vi "Grab and Attributes Setup.vi"() -> ()   [LabVIEW 2011]
doc: "The Grab and Attributes Setup example VI allows the user to view the current attributes and settings, update attribute settings, acquire images continuously, and display the images in an image control."
uses:
  <vilib>/vision/driver/NI_Vision_Acquisition_Software.lvlib
  <vilib>/vision/driver/IMAQdx.llb/IMAQdx Acquisition Mode.ctl
  <vilib>/vision/driver/IMAQdx.llb/IMAQdx Buffer Number Mode.ctl
panel:
  in  "Tab Control":T1(tab)
  in  "U32 Value Control":u32(slide) scale=0.0..4047.0
  in  "DBL Value Control":dbl(slide) min=1e-06 max=1000.0 step=1.0 scale=1e-06..1000.0
  in  "String Value Control":string
  in  "Enum Value Control":u32(ring) items=["Red", "Green", "Blue"]
  in  "Boolean Value Control":bool
  in  "Command Value Control":bool
  in  "Grab":bool
  out "Tooltip":string
  out "Units":string
  in  "Attribute Tree":string(tree)
  out "Frame Rate":dbl(knob) scale=0.0..100.0
  out "Image":T2(plugin-control)
  out "Buffer Number":u32
  in  "Camera Name":refnum<k21> caption="IMAQdx Session"
  in  "Stop":bool
  # "Overview: Demonstrates how to view the current attributes and settings, update attribute settings, acquire images continuously, and display the images in an image control.\nRequirements: Vision Acquisition Software\nInstructions: \n1. Select the Camera Name\n2. Run the VI"
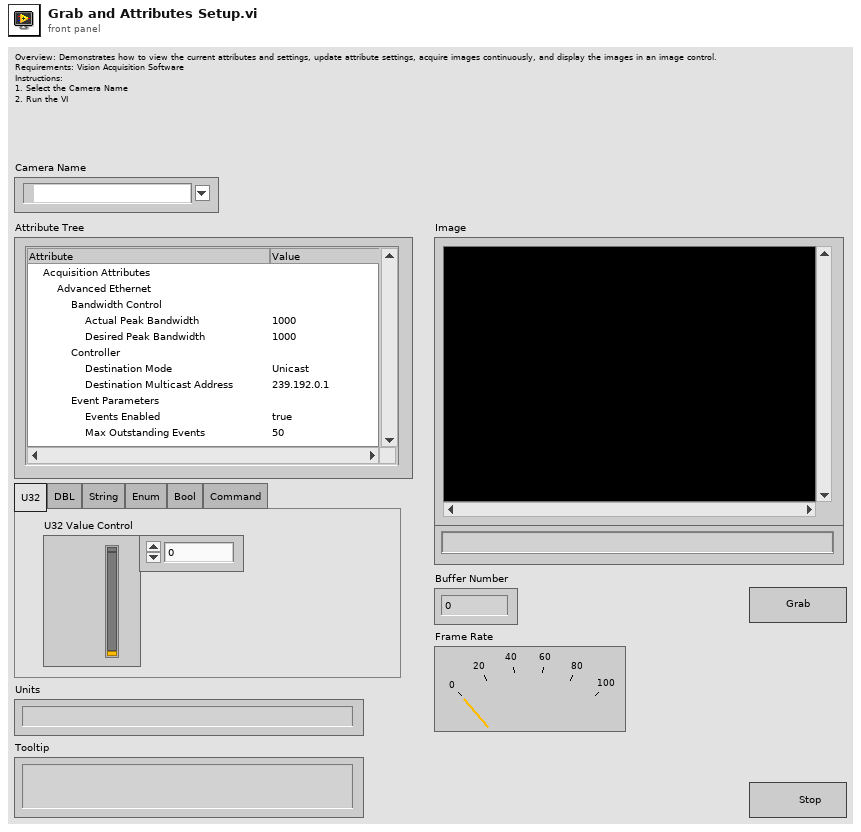
[diagram p1: front panel]
types:
  T1 = enum32{"U32", "DBL", "String", "Enum", "Bool", "Command"}
  T2 = typedef "IMAQ Image.ctl" = refnum<image>
  T3 = typedef "NI_Vision_Acquisition_Software.lvlib/IMAQdx Acquisition Mode.ctl" = enum32{"One Shot", "Continuous"}
  T4 = typedef "IMAQdx.ctl" = refnum<k21>
  T5 = cluster{"Tab Control":refnum<vi>, "U32 Value Control":refnum<vi>, "DBL Value Control":refnum<vi>, "String Value Control":refnum<vi>, "Enum Value Control":refnum<vi>, "Boolean Value Control":refnum<vi>, "Command Value Control":refnum<vi>}
  T6 = typedef "NI_Vision_Acquisition_Software.lvlib/IMAQdx Buffer Number Mode.ctl" = enum32{"Next", "Last", "Buffer Number", "Every", "Last New"}
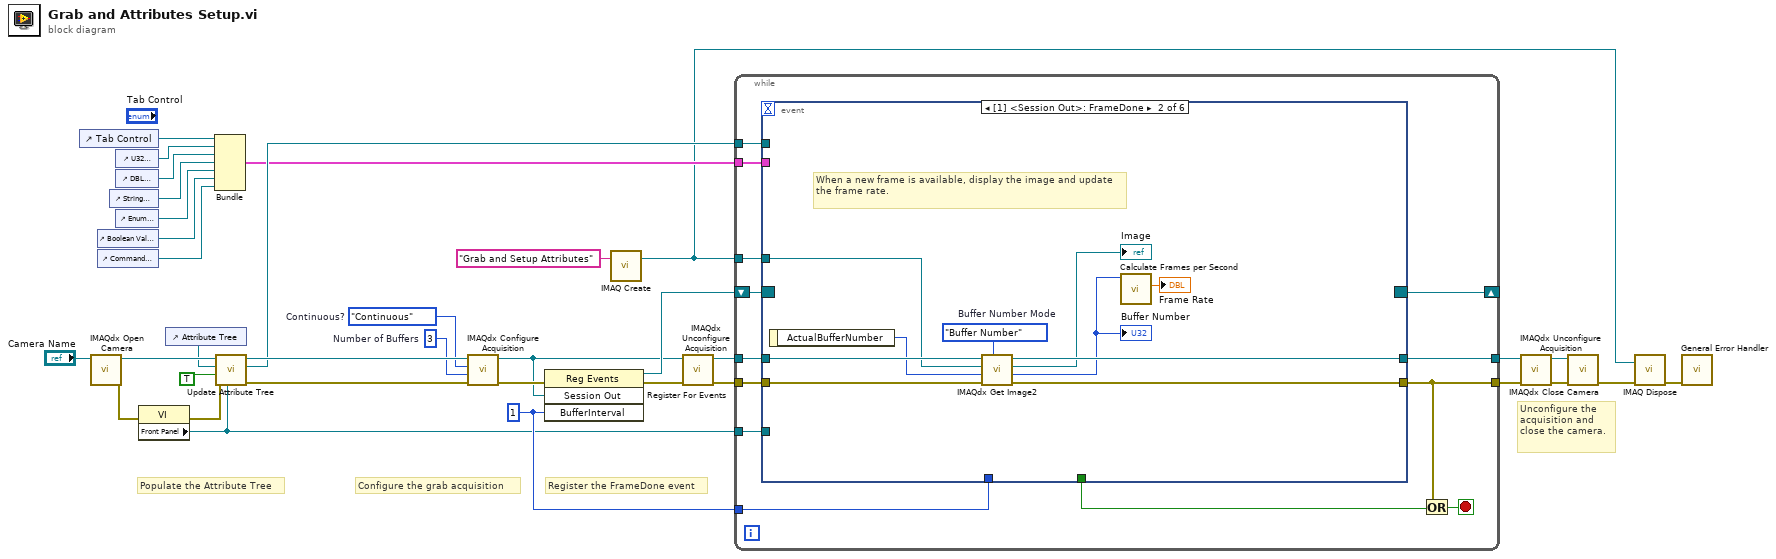
[diagram p0: block diagram]
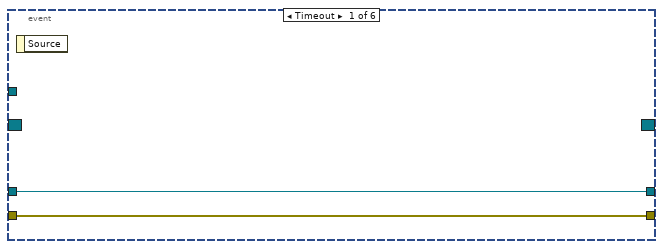
[diagram p2: hidden frame]
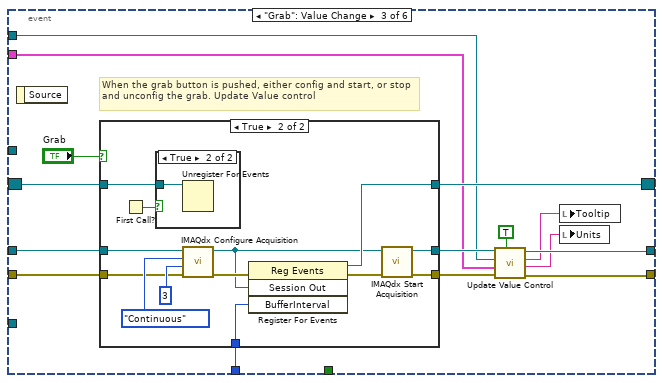
[diagram p3: hidden frame]
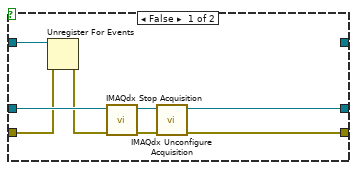
[diagram p4: hidden frame]
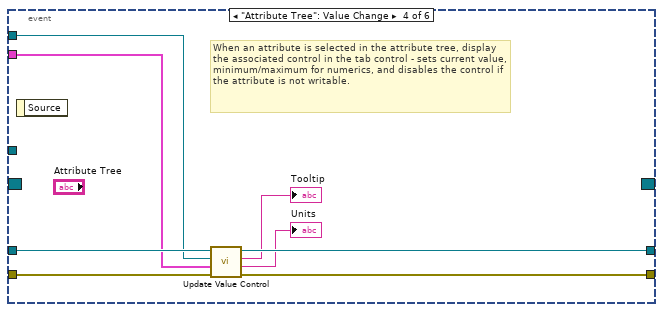
[diagram p6: hidden frame]
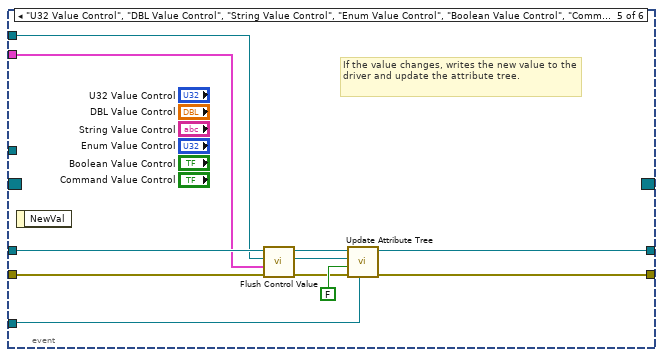
[diagram p7: hidden frame]
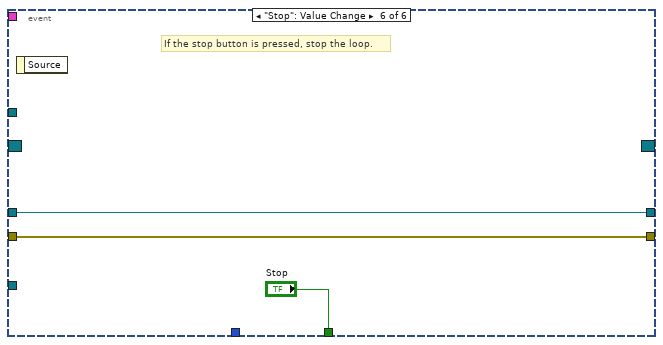
[diagram p8: hidden frame]
diagram:
  w16 = u32 1 ("BufferInterval")
  w2 = u32 3  # Number of Buffers
  w1 = IMAQdx_Acquisition_Mode."Continuous"  # Continuous?
  # "Unconfigure the acquisition and close the camera."
  # "Register the FrameDone event"
  # "Configure the grab acquisition"
  # "Populate the Attribute Tree"
  n1 = control-ref of="Tab Control"() -> (w6:refnum<vi>)
  n2 = call <vilib>:"IMAQdx Open Camera.vi"("Session In"="Camera Name") -> ("error out"=w19:errorcluster, "Session Out"=w24:T4)  [unwired: 2 in, 7 out]
  n3 = control-ref of="Boolean Value Control"() -> (w26:refnum<vi>)
  n4 = control-ref of="Command Value Control"() -> (w25:refnum<vi>)
  n5 = control-ref of="String Value Control"() -> (w30:refnum<vi>)
  n6 = control-ref of="U32 Value Control"() -> (w29:refnum<vi>)
  n7 = control-ref of="DBL Value Control"() -> (w28:refnum<vi>)
  n8 = control-ref of="Enum Value Control"() -> (w27:refnum<vi>)
  n9 = property class="VI"(error in=w19) -> (error out=w5:errorcluster, "Front Panel"=w3:refnum<vi>)  [unwired: 1 in, 1 out]
  n10 = control-ref of="Attribute Tree"() -> (w22:refnum<vi>)
  n11 = Bundle("Tab Control"=w6, "U32 Value Control"=w29, "DBL Value Control"=w28, "String Value Control"=w30, "Enum Value Control"=w27, "Boolean Value Control"=w26, "Command Value Control"=w25) -> (w11:T5)  [unwired: 1 out]
  n12 = call "Update Attribute Tree.vi"("Panel Refnum In"=w3, "error in"=w5, "Flush Tree?"=TRUE, "Tree Control In"=w22, "Camera Name In"=w24) -> ("error out"=w4:errorcluster, "Tree Control Out"=w20:refnum<vi>, "Session Out"=w23:T4)  [unwired: 4 in]
  n13 = call <vilib>:"IMAQdx Configure Acquisition.vi"("error in"=w4, "Number of Buffers"=w2, "Continuous?"=w1, "Session In"=w23) -> ("error out"=w32:errorcluster, "Session Out"=w13:T4)  [unwired: 6 out]
  n14 = register-events(error in=w32, w13, w16) -> (reference out=w31:refnum<event-registration>, error out=w15:errorcluster)  [unwired: 1 in]
  n15 = call "IMAQ Create"("Image Name"="Grab and Setup Attributes") -> ("New Image"=w8:T2)  [unwired: 3 in, 2 out]
  n16 = call <vilib>:"IMAQdx Unconfigure Acquisition.vi"("error in"=w15, "Session In"=w13) -> ("error out"=w14:errorcluster, "Session Out"=w12:T4)  [unwired: 8 out]
  n17 = while {
    tunnel: [w44] -> w18
    tunnel: w14 -> [w46]
    tunnel: w12 -> [w47]
    tunnel: [w37] -> w17
    tunnel: w8 -> [w45]
    tunnel: w20 -> [w42]
    tunnel: w3 -> [w41]
    tunnel: w16 -> [w39]
    shift-right: [w38] -> _
    shift-left: w31 -> [w43]
    tunnel: w11 -> [w36]
    stop <- w48 stop-if-true
    n18 = event shown="[1] <Session Out>: FrameDone" {
      selector: w43 -> [_ _ w71 _ _ _]
      dyn-events: [_ _ w73 _ _ _] -> w38
      timeout: _ -> [_ _ _ _ _ _]
      tunnel: w47 -> [w49 w60 w75 w105 w115 w117]
      tunnel: w46 -> [w50 w59 w70 w103 w116 w118]
      tunnel: w45 -> [_ w58 _ _ _ _]
      tunnel: [w49 w57 w63 w104 w111 w117] -> w44
      tunnel: [w50 w56 w67 w102 w107 w118] -> w37
      tunnel: w42 -> [_ _ w66 w100 w109 _]
      tunnel: w41 -> [_ _ _ _ w106 _]
      tunnel: [_ _ _ _ _ "Stop"] -> w40
      tunnel: w39 -> [_ _ w72 _ _ _]
      tunnel: w36 -> [_ _ w64 w101 w110 _]
      event Timeout {
        n19 = event-data() -> ()  [unwired: 2 out]
      }
      event event #0x0 {
        w54 = IMAQdx_Buffer_Number_Mode."Buffer Number"  # Buffer Number Mode
        # "When a new frame is available, display the image and update the frame rate."
        n20 = event-data() -> ("ActualBufferNumber"=w53:u32)  [unwired: 1 out]
        n21 = call <vilib>:"IMAQdx Get Image2.vi"("Buffer Number Mode (Next)"=w54, "error in"=w59, "Buffer Number In"=w53, "Image In"=w58, "Session In"=w60) -> ("error out"=w56:errorcluster, "Buffer Number Out"=w52:u32, "Image Out"=→"Image":T2, "Session Out"=w57:T4)  [unwired: 3 in]
        "Buffer Number" <- w52
        n22 = call <vilib>:"Calculate Frames per Second.vi"("Buffer Number"=w52) -> ("Processed Frames/s"=→"Frame Rate":dbl)  [unwired: 8 in, 2 out]
      }
      event "Grab": Value Change {
        # "When the grab button is pushed, either config and start, or stop and unconfig the grab. Update Value control"
        n23 = event-data() -> ()  [unwired: 2 out]
        n24 = case shown="True" "Grab" {
          tunnel: w75 -> [w83 w94]
          tunnel: [w80 w96] -> w69
          tunnel: [w79 w95] -> w68
          tunnel: [_ w89] -> w73
          tunnel: w72 -> [_ w87]
          tunnel: w71 -> [w78 w85]
          tunnel: w70 -> [w76 w86]
          frame False {
            n25 = Unregister For Events(event registration refnum=w78, error in=w76) -> (error out=w77:errorcluster)
            n26 = call <vilib>:"IMAQdx Stop Acquisition.vi"("error in"=w77, "Session In"=w83) -> ("error out"=w81:errorcluster, "Session Out"=w82:T4)  [unwired: 8 out]
            n27 = call <vilib>:"IMAQdx Unconfigure Acquisition.vi"("error in"=w81, "Session In"=w82) -> ("error out"=w79:errorcluster, "Session Out"=w80:T4)  [unwired: 8 out]
          }
          frame True {
            n28 = First Call?() -> (First Call?: T/F=w84:bool)
            n29 = case shown="True" w84 {
              tunnel: w85 -> [_ w97]
              frame False {
              }
              frame True {
                n30 = Unregister For Events(event registration refnum=w97) -> ()  [unwired: 1 in, 1 out]
              }
            }
            n31 = call <vilib>:"IMAQdx Configure Acquisition.vi"("error in"=w86, "Number of Buffers"=u32 3, "Continuous?"=IMAQdx_Acquisition_Mode."Continuous", "Session In"=w94) -> ("error out"=w91:errorcluster, "Session Out"=w88:T4)  [unwired: 6 out]
            n32 = register-events(error in=w91, w88, w87) -> (reference out=w89:refnum<event-registration>, error out=w90:errorcluster)  [unwired: 1 in]
            n33 = call <vilib>:"IMAQdx Start Acquisition.vi"("error in"=w90, "Session In"=w88) -> ("error out"=w95:errorcluster, "Session Out"=w96:T4)  [unwired: 8 out]
          }
        }
        n34 = call "Update Value Control.vi"("Force update?"=TRUE, "error in (no error)"=w68, "Tab Control Ref In"=w64, "Tree Control In"=w66, "Session In"=w69) -> ("error out"=w67:errorcluster, "Units"=w61:string, "Tooltip"=w62:string, "Session Out"=w63:T4)  [unwired: 3 in]
        n35 = local write "Tooltip"(w62) -> ()
        n36 = local write "Units"(w61) -> ()
      }
      event "Attribute Tree": Value Change {
        # "When an attribute is selected in the attribute tree, display the associated control in the tab control - sets current value, minimum/maximum for numerics, and disables the control if the attribute is not writable."
        n37 = event-data() -> ()  [unwired: 2 out]
        n38 = call "Update Value Control.vi"("error in (no error)"=w103, "Tab Control Ref In"=w101, "Tree Control In"=w100, "Session In"=w105) -> ("error out"=w102:errorcluster, "Units"=→"Units":string, "Tooltip"=→"Tooltip":string, "Session Out"=w104:T4)  [unwired: 4 in]
      }
      event "U32 Value Control", "DBL Value Control", "String Value Control", "Enum Value Control", "Boolean Value Control", "Command Value Control": Value Change {
        # "If the value changes, writes the new value to the driver and update the attribute tree."
        n39 = event-data() -> ()  [unwired: 2 out]
        n40 = call "Flush Control Value.vi"("error in (no error)"=w116, "Tab Control Ref In"=w110, "Tree Control In"=w109, "Session In"=w115) -> ("error out"=w108:errorcluster, "Tree Control Out"=w113:refnum<vi>, "Session Out"=w114:T4)  [unwired: 5 in]
        n41 = call "Update Attribute Tree.vi"("Panel Refnum In"=w106, "error in"=w108, "Flush Tree?"=FALSE, "Tree Control In"=w113, "Camera Name In"=w114) -> ("error out"=w107:errorcluster, "Session Out"=w111:T4)  [unwired: 4 in, 1 out]
      }
      event "Stop": Value Change {
        # "If the stop button is pressed, stop the loop."
        n42 = event-data() -> ()  [unwired: 2 out]
      }
    }
    n43 = Or(x=w37, y=w40) -> (x .or. y?=w48:bool)
  }
  n44 = call <vilib>:"IMAQdx Unconfigure Acquisition.vi"("error in"=w17, "Session In"=w18) -> ("error out"=w34:errorcluster, "Session Out"=w33:T4)  [unwired: 8 out]
  n45 = call <vilib>:"IMAQdx Close Camera.vi"("error in"=w34, "Session In"=w33) -> ("error out"=w10:errorcluster)  [unwired: 9 out]
  n46 = call "IMAQ Dispose"("Image"=w8, "error in (no error)"=w10) -> ("error out"=w9:errorcluster)  [unwired: 4 in]
  n47 = call <vilib>:"General Error Handler.vi"("error in (no error)"=w9) -> ()  [unwired: 1 in, 14 out]
